vi "PPR_SIM_SIM_WHEEL_INIT.vi"(3 "Side":string, 5 "Drive PWM Channel":T2, 6 "DriveDistPerCount":dbl=1.0, 10 "Drive B Channel":T1, 11 "Drive A channel":T1) -> ()   [LabVIEW 2019]
uses:
  <vilib>/Rock Robotics/SystemInterfaces/DIO/FPGA_DIOPWMChannel.ctl
  <vilib>/Rock Robotics/SystemInterfaces/DIO/FPGA_DIOChannel.ctl
  PPR_SIM_SIM_Globals.vi
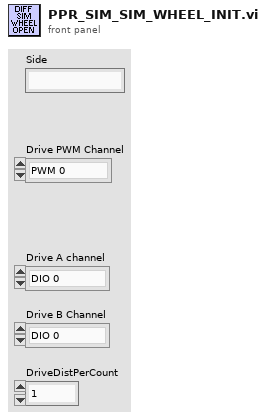
[diagram p1: front panel]
types:
  T1 = typedef "FPGA_DIOChannel.ctl" = enum8{"DIO 0", "DIO 1", "DIO 2", "DIO 3", "DIO 4", "DIO 5", "DIO 6", "DIO 7", "DIO 8", "DIO 9", "DIO MXP 0", "DIO MXP 1", "DIO MXP 2", "DIO MXP 3", "DIO MXP 4", "DIO MXP 5", "DIO MXP 6", "DIO MXP 7", "DIO MXP 8", "DIO MXP 9", "DIO MXP 10", "DIO MXP 11", "DIO MXP 12", "DIO MXP 13", "DIO MXP 14", "DIO MXP 15", "SPI Port CS1", "SPI Port CS2", "SPI Port CS3", "SPI Port MISO", "SPI Port MOSI", "Invalid"}
  T2 = typedef "FPGA_DIOPWMChannel.ctl" = enum8{"PWM 0", "PWM 1", "PWM 2", "PWM 3", "PWM 4", "PWM 5", "PWM 6", "PWM 7", "PWM 8", "PWM 9", "PWM MXP 0", "PWM MXP 1", "PWM MXP 2", "PWM MXP 3", "PWM MXP 4", "PWM MXP 5", "PWM MXP 6", "PWM MXP 7", "PWM MXP 8", "PWM MXP 9", "Invalid"}
  T3 = cluster{"Diff Motor Device Index":i32, "Wheel Encoder Device Index":i32, "Wheel DistPerzcount":dbl}[]
  T4 = typedef "PPR_DRIVE_Wheel_TYPDEF.ctl" = cluster{"Drive Motor":T5, "Wheel Encoder":T8}
  T5 = typedef "WPI_MotorControlDeviceRef.ctl" = cluster{"DeviceStatus":errorcluster, "Type":T6, "PWM":cluster{"PWM Channel":T2, "DeadBand":T7}, "CAN":cluster{"Device Number":u8, "SetOutput VI Ref":variant, "GetOutput VI Ref":variant, "Enable VI Ref":variant, "Disable VI Ref":variant, "Data":variant}, "Invert":bool, "DIO PWM":cluster{"PWM \"Enable\" Channel":T2, "DIOChannel":T1, "PWM Rate":dbl}}
  T6 = typedef "WPI_MotorControlType.ctl" = enum16{"PWM", "CAN", "DIO PWM"}
  T7 = typedef "WPI_PWMDeadband.ctl" = cluster{"Name":string, "maxPositivePwm":i32, "minPositivePwm":i32, "centerPwm":i32, "maxNegativePwm":i32, "minNegativePwm":i32, "angularRange":u16}
  T8 = typedef "WPI_EncoderDevRef.ctl" = cluster{"DevStatus":errorcluster, "EncoderIndex":T9, "CounterIndex":T10, "DistancePerCount":dbl, "Decoding Type":T11}
  T9 = typedef "FPGA_EncoderIdx.ctl" = enum8{"Enc 0", "Enc 1", "Enc 2", "Enc 3", "Enc 4", "Enc 5", "Enc 6", "Enc 7", "Invalid"}
  T10 = typedef "FPGA_CounterCtrSystemIndex.ctl" = enum8{"Ctr 0", "Ctr 1", "Ctr 2", "Ctr 3", "Ctr 4", "Ctr 5", "Ctr 6", "Ctr 7", "Invalid"}
  T11 = typedef "WPI_EncoderType.ctl" = enum16{"1x", "2x", "4x"}
  T12 = cluster{"Diff Motor Device Index":i32, "Wheel Encoder Device Index":i32, "Wheel DistPerzcount":dbl}
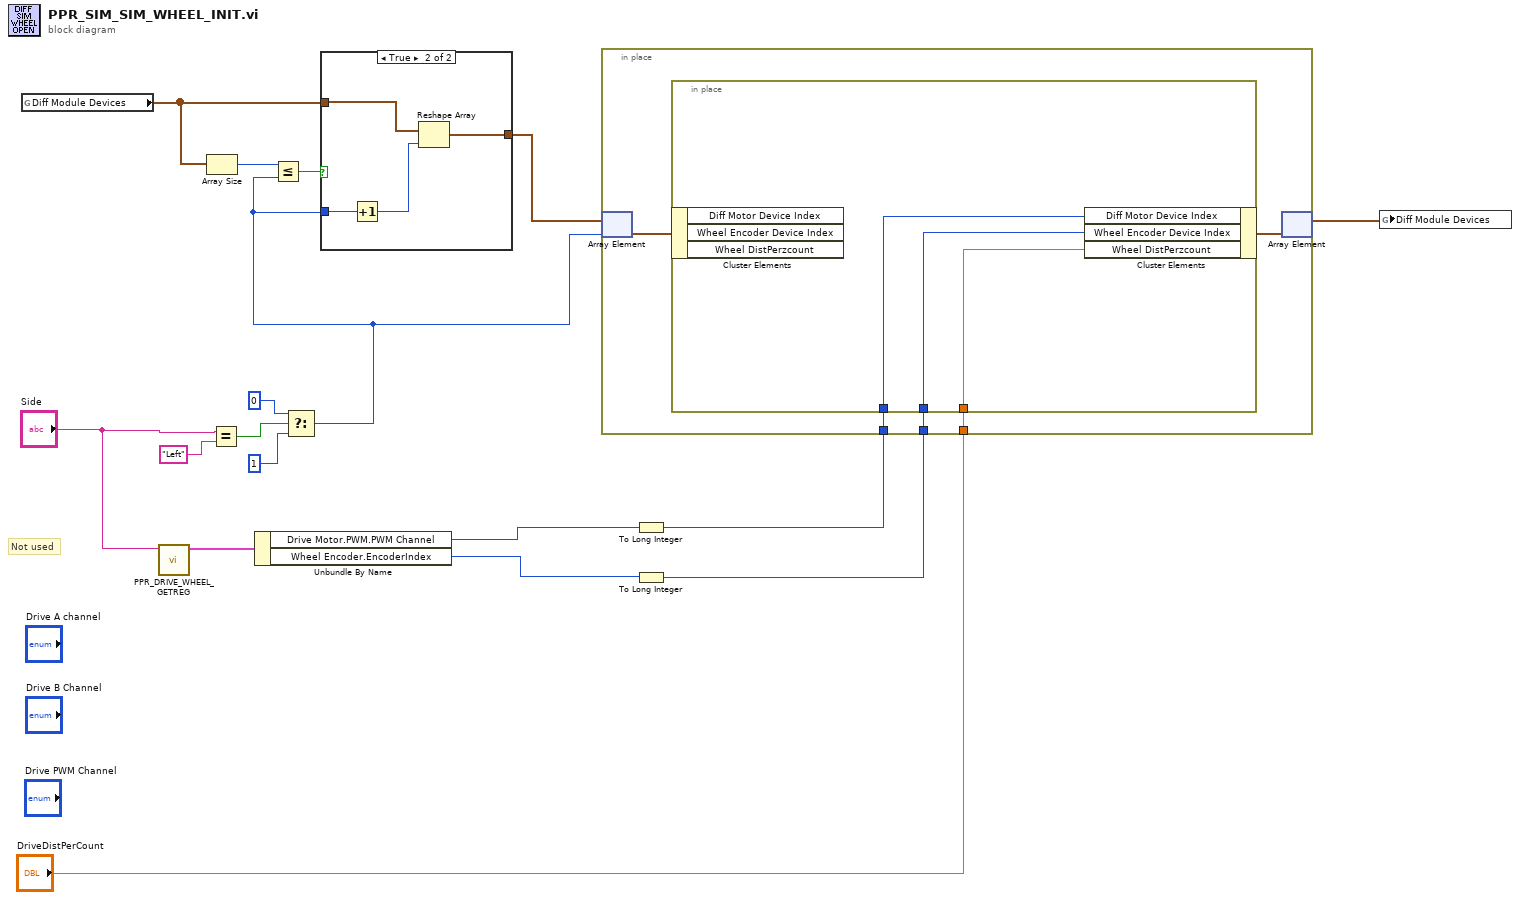
[diagram p0: block diagram]
diagram:
  # "Not used"
  n1 = global read "PPR_SIM_SIM_Globals.vi" "Diff Module Devices"() -> (w13:T3)
  n2 = call "PPR_DRIVE_WHEEL_GETREG.vi"("Side"="Side") -> ("Diff Wheel TypDef"=w11:T4)  [unwired: 10 in]
  n3 = Array Size(array=w13) -> (size(s)=w15:i32)
  n4 = Equal?(x="Side", y="Left") -> (x = y?=w8:bool)
  n5 = Unbundle By Name(w11) -> ("Drive Motor.PWM.PWM Channel"=w10:T2, "Wheel Encoder.EncoderIndex"=w3:T9)
  n6 = Select(t=0, s=w8, f=1) -> (s? t:f=w4:i32)
  n7 = Less Or Equal?(x=w15, y=w4) -> (x <= y?=w14:bool)
  n8 = case shown="True" w14 {
    tunnel: w13 -> [w18 w20]
    tunnel: w4 -> [_ w22]
    tunnel: [w18 w19] -> w12
    frame False {
    }
    frame True {
      n9 = Increment(x=w22) -> (x+1=w21:i32)
      n10 = Reshape Array(w20, w21) -> (w19:T3)
    }
  }
  n11 = To Long Integer(number=w10) -> (32bit integer=w16:i32)
  n12 = To Long Integer(number=w3) -> (32bit integer=w2:i32)
  n13 = in-place {
    in-place-border: w16 -> [w26]
    in-place-border: w2 -> [w24]
    in-place-border: "DriveDistPerCount" -> [w23]
    n14 = in-place-array #1(w12, w4) -> (w27:T12)
    n15 = in-place {
      in-place-border: w26 -> [w30]
      in-place-border: w24 -> [w29]
      in-place-border: w23 -> [w28]
      n16 = in-place-cluster #2(w27) -> ()  [unwired: 3 out]
      n17 = in-place-cluster #2("Diff Motor Device Index"=w30, "Wheel Encoder Device Index"=w29, "Wheel DistPerzcount"=w28) -> (w25:T12)
    }
    n18 = in-place-array #1(w25) -> (w17:T3)  [unwired: 1 out]
  }
  n19 = global write "PPR_SIM_SIM_Globals.vi" "Diff Module Devices"(w17) -> ()
